vi "main_panel_run_init.vi"(3 "Env ready?":refnum<vi>) -> (0 "Cancelled?":bool)   [LabVIEW 2019]
uses:
  lib/libSimulationControl/libSimulationControl.lvlib
panel:
  # "*******************************************************************\nBiogas Plant Control\n\nAuthor: Paul Zügel\nGCSC-Frankfurt am Main 2020\n\n*******************************************************************"
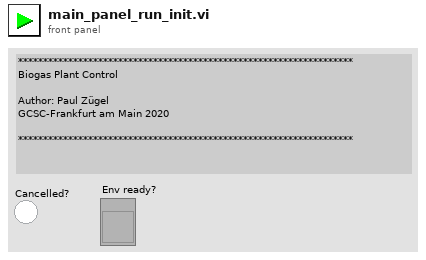
[diagram p1: front panel]
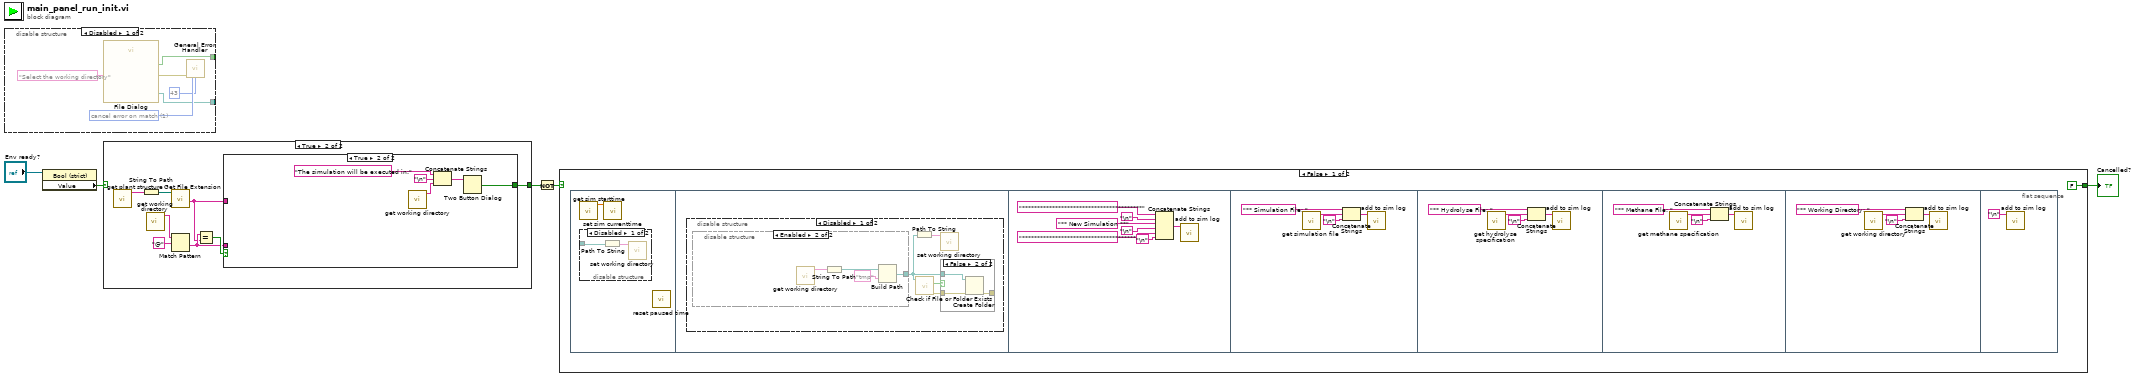
[diagram p0: block diagram]
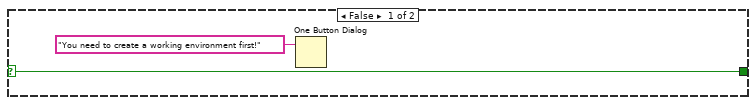
[diagram p2: hidden frame]
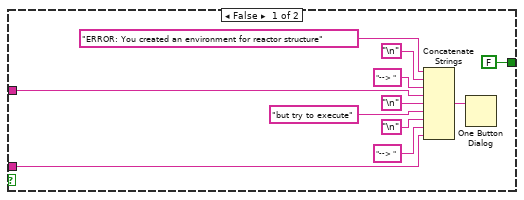
[diagram p3: hidden frame]
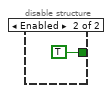
[diagram p4: hidden frame]
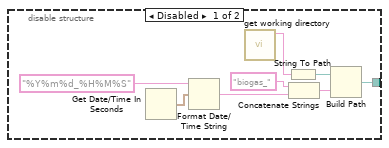
[diagram p6: hidden frame]
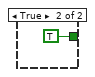
[diagram p9: hidden frame]
diagram:
  n1 = disable-structure shown="Disabled" {
    disable-tunnel: [w8 TRUE ("cancelled")] -> _
    disable-tunnel: [w6 _] -> _
    frame Disabled {
      w10 = 1 items=["no exception", "cancel error on match", "set error on match"] ("[exception action] (none:0)")
      n2 = call "File Dialog"("prompt"="Select the working directory") -> ("selected path"=w6:path, "cancelled"=w8:bool, "error out"=w11:errorcluster)  [unwired: 11 in, 1 out]
      n3 = call <vilib>:"General Error Handler.vi"("error in (no error)"=w11, "[exception action] (none:0)"=w10, "[exception code]"=43) -> ()  [unwired: 8 in, 5 out]
    }
    frame Enabled {
    }
  }
  n4 = property on="Property Node" class="Bool (strict)"(reference="Env ready?") -> ("Value"=w3:bool)  [unwired: 1 in, 2 out]
  n5 = case shown="True" w3 {
    selector: w3 -> [w14 _]
    tunnel: [w14 w22] -> w1
    frame False {
      n6 = One Button Dialog(message="You need to create a working environment first!") -> ()  [unwired: 1 in, 1 out]
    }
    frame True {
      n7 = call "get plant structure.vi"() -> ("function return"=w16:string)  [unwired: 10 in, 1 out]
      n8 = String To Path(string=w16) -> (path=w15:path)
      n9 = call "get working directory.vi"() -> ("function return"=w21:string)  [unwired: 10 in, 1 out]
      n10 = call <vilib>:"Get File Extension.vi"("file"=w15) -> ("filename without extension"=w17:string)  [unwired: 6 in, 4 out]
      n11 = Match Pattern(string=w21, regular expression="@") -> (after substring=w18:string)  [unwired: 1 in, 3 out]
      n12 = Equal?(x=w18, y=w17) -> (x = y?=w19:bool)
      n13 = case shown="True" w19 {
        tunnel: [FALSE ("T button?") w34] -> w22
        tunnel: w18 -> [w23 _]
        tunnel: w17 -> [w28 _]
        frame False {
          n14 = Concatenate Strings("ERROR: You created an environment for reactor structure" ("string"), "\n", "--> " ("string"), w28, "\n", "but try to execute" ("string"), "\n", "--> " ("string"), w23) -> (w32:string)
          n15 = One Button Dialog(message=w32) -> ()  [unwired: 1 in, 1 out]
        }
        frame True {
          n16 = call "get working directory.vi"() -> ("function return"=w36:string)  [unwired: 10 in, 1 out]
          n17 = Concatenate Strings("The simulation will be executed in:" ("string"), "\n", w36) -> (w35:string)
          n18 = Two Button Dialog(message=w35) -> (T button?=w34:bool)  [unwired: 2 in]
        }
      }
    }
  }
  n19 = Not(x=w1) -> (.not. x?=w2:bool)
  n20 = case shown="False" w2 {
    tunnel: [FALSE TRUE] -> w5
    frame False {
      n21 = flat-sequence {
        frame #0 {
          n22 = call "get sim starttime.vi"() -> ("sim_starttime"=w40:dbl)  [unwired: 10 in, 1 out]
          n23 = disable-structure shown="Disabled" {
            disable-tunnel: _ -> [w41 _]
            frame Disabled {
              n24 = Path To String(path=w41) -> (string=w42:string)
              n25 = call "set working directory.vi"("dir"=w42) -> ()  [unwired: 10 in, 1 out]
            }
            frame Enabled {
            }
          }
          n26 = call "set sim currenttime.vi"("time"=w40) -> ()  [unwired: 10 in, 1 out]
          n27 = call "reset paused time.vi"() -> ()  [unwired: 11 in, 1 out]
        }
        frame #1 {
          n28 = disable-structure shown="Disabled" {
            frame Disabled {
              n29 = disable-structure shown="Enabled" {
                disable-tunnel: [w54 w57] -> w46
                frame Disabled {
                  n30 = Get Date/Time In Seconds() -> (seconds since 1Jan1904=w51:timestamp)
                  n31 = Format Date/Time String(time format string (%c)="%Y%m%d_%H%M%S", seconds (now)=w51) -> (date/time string=w52:string)  [unwired: 1 in]
                  n32 = call "get working directory.vi"() -> ("function return"=w48:string)  [unwired: 10 in, 1 out]
                  n33 = String To Path(string=w48) -> (path=w47:path)
                  n34 = Concatenate Strings("biogas_" ("string"), w52) -> (w53:string)
                  n35 = Build Path(base path=w47, name or relative path=w53) -> (appended path=w54:path)
                }
                frame Enabled {
                  n36 = call "get working directory.vi"() -> ("function return"=w55:string)  [unwired: 10 in, 1 out]
                  n37 = String To Path(string=w55) -> (path=w56:path)
                  n38 = Build Path(base path=w56, name or relative path="tmp") -> (appended path=w57:path)
                }
              }
              n39 = Path To String(path=w46) -> (string=w44:string)
              n40 = call <vilib>:"Check if File or Folder Exists.vi"("path"=w46) -> ("error out"=w45:errorcluster, "file or folder exists?"=w43:bool)  [unwired: 8 in, 1 out]
              n41 = call "set working directory.vi"("dir"=w44) -> ()  [unwired: 10 in, 1 out]
              n42 = case shown="False" w43 {
                tunnel: w46 -> [_ w62]
                tunnel: [w59 w61] -> _
                tunnel: w45 -> [w59 w60]
                frame True {
                }
                frame False {
                  n43 = Create Folder(path (use dialog)=w62, error in=w60) -> (error out=w61:errorcluster)  [unwired: 1 in, 2 out]
                }
              }
            }
            frame Enabled {
            }
          }
        }
        frame #2 {
          n44 = Concatenate Strings("****************************************" ("string"), "\n", "** New Simulation **" ("string"), "\n", "****************************************" ("string"), "\n") -> (w69:string)
          n45 = call "add to sim log.vi"("log"=w69) -> ()  [unwired: 10 in, 1 out]
        }
        frame #3 {
          n46 = call "get simulation file.vi"() -> ("function return"=w73:string)  [unwired: 10 in, 1 out]
          n47 = Concatenate Strings("** Simulation File: " ("string"), w73, "\n") -> (w72:string)
          n48 = call "add to sim log.vi"("log"=w72) -> ()  [unwired: 10 in, 1 out]
        }
        frame #4 {
          n49 = call "get hydrolyse specification.vi"() -> ("function return"=w74:string)  [unwired: 10 in, 1 out]
          n50 = Concatenate Strings("** Hydrolyse File: " ("string"), w74, "\n") -> (w77:string)
          n51 = call "add to sim log.vi"("log"=w77) -> ()  [unwired: 10 in, 1 out]
        }
        frame #5 {
          n52 = call "get methane specification.vi"() -> ("function return"=w78:string)  [unwired: 10 in, 1 out]
          n53 = Concatenate Strings("** Methane File: " ("string"), w78, "\n") -> (w81:string)
          n54 = call "add to sim log.vi"("log"=w81) -> ()  [unwired: 10 in, 1 out]
        }
        frame #6 {
          n55 = call "get working directory.vi"() -> ("function return"=w85:string)  [unwired: 10 in, 1 out]
          n56 = Concatenate Strings("** Working Directory: " ("string"), w85, "\n") -> (w84:string)
          n57 = call "add to sim log.vi"("log"=w84) -> ()  [unwired: 10 in, 1 out]
        }
        frame #7 {
          n58 = call "add to sim log.vi"("log"="\n") -> ()  [unwired: 10 in, 1 out]
        }
      }
    }
    frame True {
    }
  }
  "Cancelled?" <- w5
